vi "GetReadmeHTML.vi"(4 "Element":string="user-content-release-notes-for-vip-packages", 5 "URL":string="https://api.github.com/repos/labviewforRaspi/LabVIEWforRasPi/contents/README.md?ref=master", 6 "error in":errorcluster, 9 "WebBrowser in":refnum<k24>) -> (0 "error out":errorcluster, 3 "WebBrowser out":refnum<k24>)   [LabVIEW 2014, in "Raspberry Pi Compatible Compiler for LabVIEW.lvlib" / "GitHub API.lvlib"]
uses:
  GitHub API.lvlib
  System.Windows.Forms
  <vilib>/httpClient/LabVIEWHTTPClient.lvlib
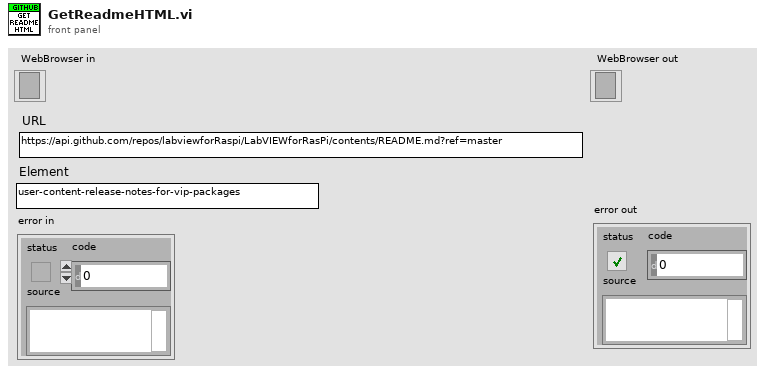
[diagram p1: front panel]
types:
  T1 = typedef "LabVIEWHTTPClient.lvlib/ClientHandle.ctl" = refnum<k1>
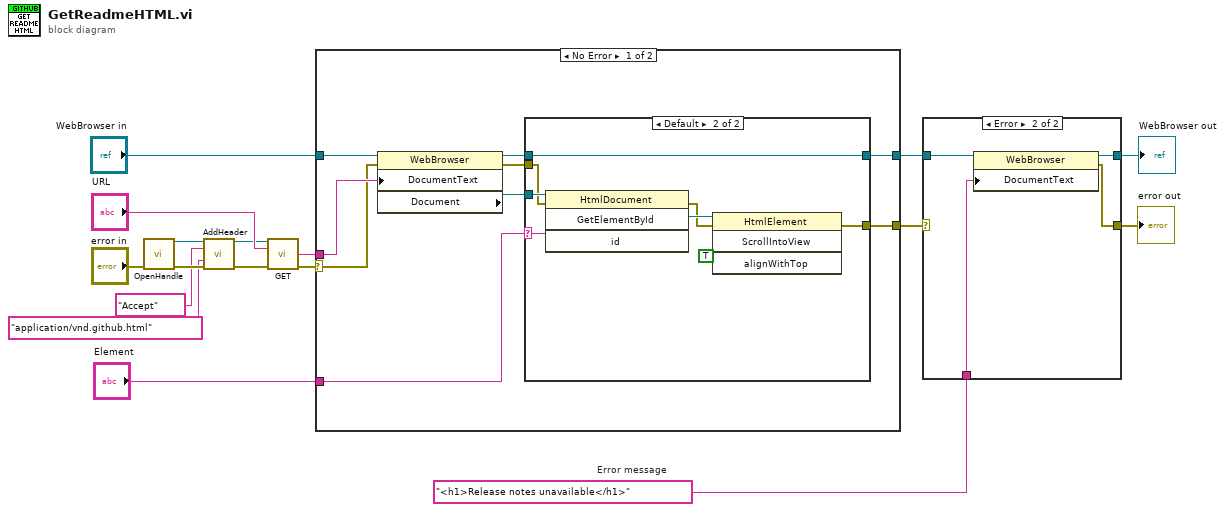
[diagram p0: block diagram]
diagram:
  w1 = "<h1>Release notes unavailable</h1>"  # Error message
  n1 = call <vilib>:"OpenHandle.vi"("error in (no error)"="error in") -> ("client handle out"=w16:T1, "error out"=w15:errorcluster)  [unwired: 13 in]
  n2 = call <vilib>:"AddHeader.vi"("client handle"=w16, "header"="Accept", "value"="application/vnd.github.html", "error in (no error)"=w15) -> ("client handle out"=w11:T1, "error out"=w10:errorcluster)  [unwired: 10 in]
  n3 = call <vilib>:"GET.vi"("client handle"=w11, "url"="URL", "error in (no error)"=w10) -> ("body"=w17:string, "error out"=w4:errorcluster)  [unwired: 9 in, 2 out]
  n4 = case shown="No Error" w4 {
    selector: w4 -> [w18 w38]
    tunnel: w17 -> [w26 _]
    tunnel: "WebBrowser in" -> [w24 w37]
    tunnel: "Element" -> [w22 _]
    tunnel: [w20 w38] -> w6
    tunnel: [w19 w37] -> w5
    frame No Error {
      n5 = property class="WebBrowser"(reference=w24, error in=w18, "DocumentText"=w26) -> (reference out=w21:refnum<k24>, error out=w23:errorcluster, "Document"=w25:refnum<k24>)
      n6 = case shown="Default" w22 {
        selector: w22 -> [_ w33]
        tunnel: w25 -> [_ w36]
        tunnel: w23 -> [w28 w35]
        tunnel: [w28 w34] -> w20
        tunnel: w21 -> [w27 w32]
        tunnel: [w27 w32] -> w19
        frame "" {
        }
        frame Default {
          n7 = invoke class="HtmlDocument" method="GetElementById"(reference=w36, error in=w35, "id"=w33) -> (error out=w29:errorcluster, "GetElementById"=w30:refnum<k24>)  [unwired: 1 in, 2 out]
          n8 = invoke class="HtmlElement" method="ScrollIntoView"(reference=w30, error in=w29, "alignWithTop"=TRUE) -> (error out=w34:errorcluster)  [unwired: 1 in, 3 out]
        }
      }
    }
    frame Error {
    }
  }
  n9 = case shown="Error" w6 {
    selector: w6 -> [w40 _]
    tunnel: w5 -> [w39 w44]
    tunnel: [w40 w42] -> w3
    tunnel: [w39 w43] -> w2
    tunnel: w1 -> [_ w41]
    frame No Error {
    }
    frame Error {
      n10 = property class="WebBrowser"(reference=w44, "DocumentText"=w41) -> (reference out=w43:refnum<k24>, error out=w42:errorcluster)  [unwired: 1 in]
    }
  }
  "error out" <- w3
  "WebBrowser out" <- w2
